vi "Rolling Average.vi"(10 "New Value":dbl, 11 "Old Array":dbl[](array[numeric])) -> (2 "Calculated Value":dbl, 3 "New Array":dbl[](array[numeric]))   [LabVIEW 2018, in "Support Library.lvlib"]
uses:
  Support Library.lvlib
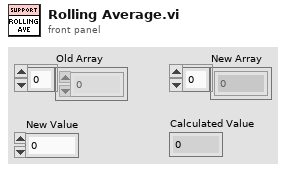
[diagram p1: front panel]
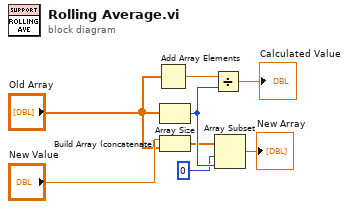
[diagram p0: block diagram]
diagram:
  n1 = Add Array Elements(numeric array="Old Array") -> (sum=w1:dbl)
  n2 = Array Size(array="Old Array") -> (size(s)=w4:i32)
  n3 = Build Array (concatenate)("New Value", "Old Array") -> (w2:dbl[])
  n4 = Divide(x=w1, y=w4) -> (x/y=→"Calculated Value":dbl)
  n5 = Array Subset(array=w2, index=0, length=w4) -> (→"New Array":dbl[])
